vi "BRig_dataMTrig_global.vi"() -> ()   [LabVIEW 2014]
panel:
  in  "dataMTrig_global":u16[](array[numeric])
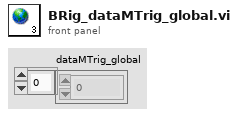
[diagram p1: front panel]
diagram:
